vi "PQ Example SELECT, Parameters.vi"() -> ()   [LabVIEW 2016]
uses:
  <vilib>/JDP Science/PostgreSQL Library/Result/PQ Result.lvclass/PQ Result.ctl
  <vilib>/JDP Science/PostgreSQL Library/Connection/Execute Command (2D string results).vi
  <vilib>/JDP Science/PostgreSQL Library/Result/Clear.vi
  <vilib>/JDP Science/PostgreSQL Library/Connection/Execute Command (Result).vi
  <vilib>/JDP Science/PostgreSQL Library/Connection/Execute (Return first result with rows).vi
  <vilib>/JDP Science/PostgreSQL Library/Connection/Single Command with parameters.vi
  <vilib>/JDP Science/PostgreSQL Library/Result/Get all results as 2D strings array.vi
  <vilib>/JDP Science/PostgreSQL Library/Connection/PQ Connection.lvclass
panel:
  in  "Connection Strings":string="host=localhost port=5433 dbname=mydb user=postgres password=******"
  in  "my_dbl Maximum":dbl=0.99 format="%#_13g"
  out "Number of Rows":i32
  out "Time per row":dbl format="%#_3p"
  out "Rows/sec":dbl format="%#_3p"
  in  "my_dbl Minimum":dbl=0.9 format="%#_13g"
  out "Strings":string[][](array[string])
  out "error out":errorcluster
  # "Run \"PQ Example Many INSERTs.vi\" first to generate data to SELCECT from"
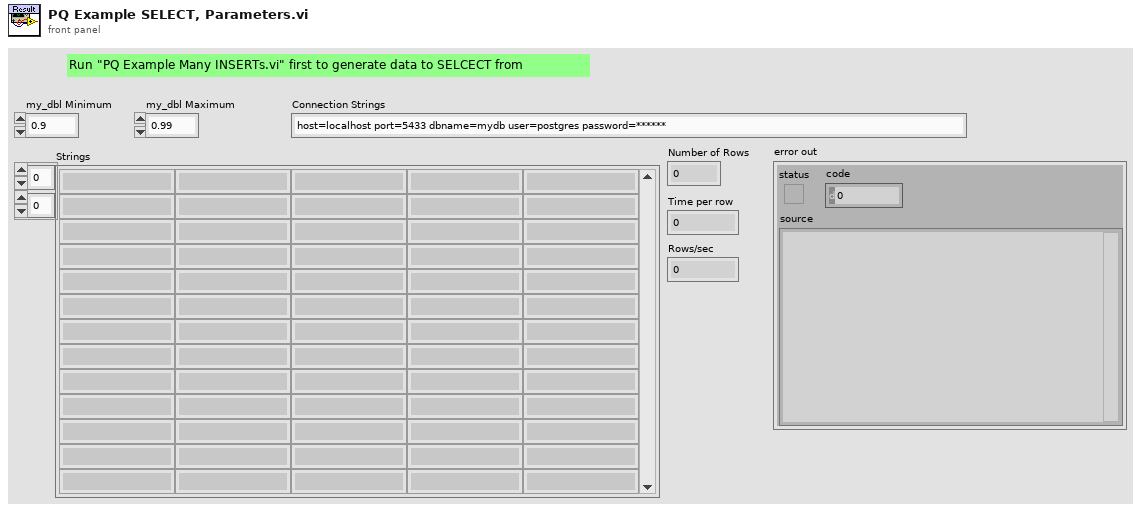
[diagram p1: front panel]
types:
  T1 = cluster{"my_dbl Minimum":dbl, "my_dbl Maximum":dbl}
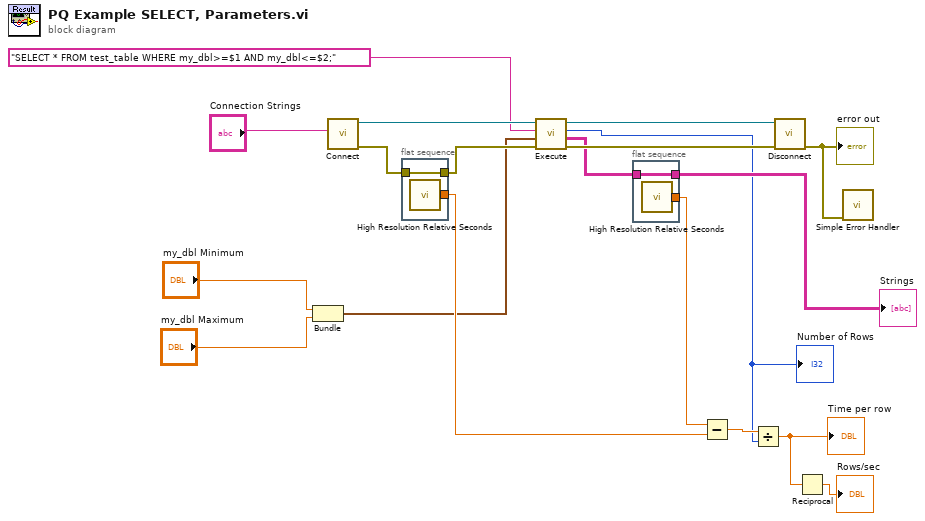
[diagram p0: block diagram]
diagram:
  n1 = Bundle("my_dbl Minimum"="my_dbl Minimum", "my_dbl Maximum"="my_dbl Maximum") -> (w1:T1)  [unwired: 1 in]
  n2 = call <vilib>:"Connect.vi"("Connection Strings"="Connection Strings") -> ("error out"=w13:errorcluster, "PQ Connection out"=w18:refnum<class "PQ Connection.lvclass">)  [unwired: 9 in]
  n3 = flat-sequence {
    tunnel: w13 -> [w21]
    tunnel: [w21] -> w12
    tunnel: [w20] -> w5
    frame #0 {
      n4 = call <vilib>:"High Resolution Relative Seconds.vi"() -> ("relative seconds"=w20:dbl)
    }
  }
  n5 = call-poly <vilib>:"Execute.vi"("error in (no error)"=w12, "Parameters"=w1, "SQL"="SELECT * FROM test_table WHERE my_dbl>=$1 AND my_dbl<=$2;" ("command"), "PQ Connection in"=w18) -> ("error out"=w15:errorcluster, "Result"=w11:string[][], "Number of Rows"=w4:i32, "PQ Connection out"=w17:refnum<class "PQ Connection.lvclass">)  [unwired: 4 in]
  "Number of Rows" <- w4
  n6 = flat-sequence {
    tunnel: w11 -> [w23]
    tunnel: [w23] -> w10
    tunnel: [w22] -> w6
    frame #0 {
      n7 = call <vilib>:"High Resolution Relative Seconds.vi"() -> ("relative seconds"=w22:dbl)
    }
  }
  n8 = Subtract(x=w6, y=w5) -> (x-y=w7:dbl)
  n9 = Divide(x=w7, y=w4) -> (x/y=w8:dbl)
  "Time per row" <- w8
  n10 = call-dynamic "Disconnect.vi"("error in (no error)"=w15, "PQ Connection in"=w17) -> ("error out"=w14:errorcluster)  [unwired: 9 in]
  "error out" <- w14
  n11 = Reciprocal(x=w8) -> (1/x=→"Rows/sec":dbl)
  n12 = call <vilib>:"Simple Error Handler.vi"("error in (no error)"=w14) -> ()  [unwired: 4 in, 5 out]
  "Strings" <- w10
